vi "str to uint32.vi"(2 "String":string) -> (6 "uint32":u32)   [LabVIEW 2013, in "OPCUA XML.lvlib"]
uses:
  OPCUA XML.lvlib
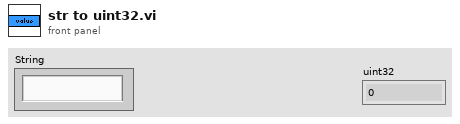
[diagram p1: front panel]
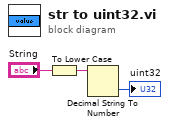
[diagram p0: block diagram]
diagram:
  n1 = To Lower Case(string="String") -> (all lower case string=w2:string)
  n2 = Decimal String To Number(string=w2) -> (number=→"uint32":i32)  [unwired: 2 in, 1 out]
